vi "SetClassInstance.vi"(11 "OsciloscopioName":string) -> (3 "specific class reference":refnum<class "Osciloscope.lvclass">)   [LabVIEW 2020]
uses:
  Classes/Implementations/Osciloscope/Osciloscope.lvclass
  Classes/Implementations/TektronicsTDS/TektroniksTDS.lvclass
  C:/Users/HP/Documents/7mo/Instrumentacion/Parcial2/Osciloscope/Osciloscopio_DuranMu-oz/OsciloscopioProject/Classes/Implementations/Osciloscope/Osciloscope.lvclass
  Classes/Implementations/Keysight/Keysight.lvclass
panel:
  out "OsciloscopeName":refnum<class "Osciloscope.lvclass">
  in  "TypeOsciloscope":string
  out "Classes":string[](array[string])
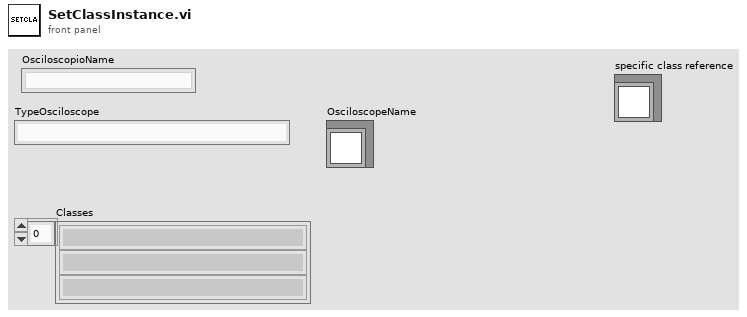
[diagram p1: front panel]
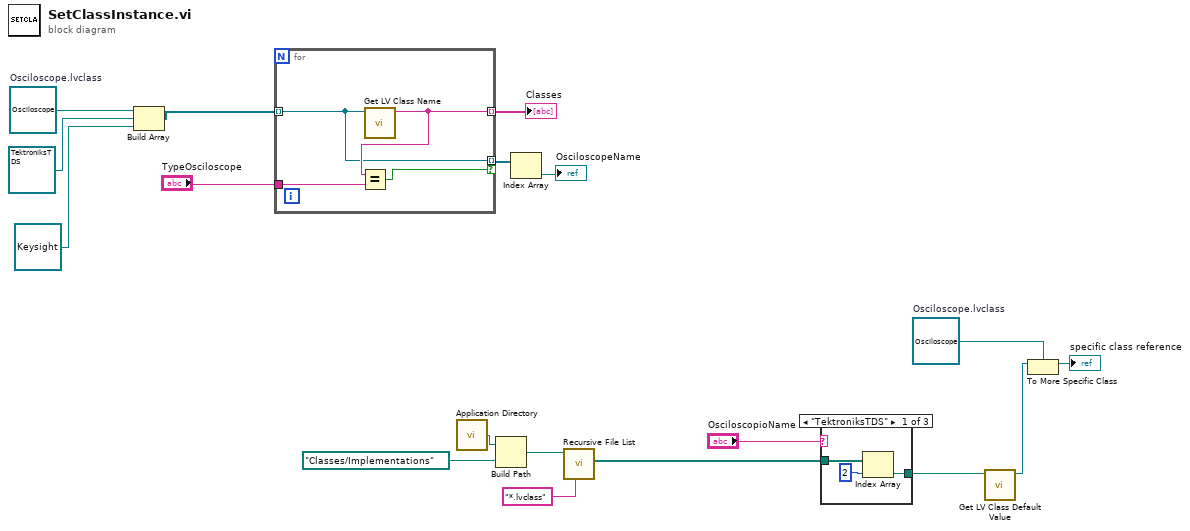
[diagram p0: block diagram]
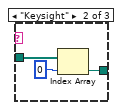
[diagram p2: hidden frame]
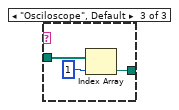
[diagram p3: hidden frame]
diagram:
  w3 = refnum<class "Osciloscope.lvclass"> refnum  # Osciloscope.lvclass
  w14 = refnum<class "Osciloscope.lvclass"> refnum  # Osciloscope.lvclass
  n1 = Build Array(w14, refnum<class "TektroniksTDS.lvclass"> refnum ("TektroniksTDS.lvclass"), refnum<class "Keysight.lvclass"> refnum ("Keysight.lvclass")) -> (w15:refnum<class "Osciloscope.lvclass">[])
  n2 = for {
    tunnel: w15 -> [w20] mode=indexing
    tunnel: [w21] -> w18 mode=indexing
    tunnel: "TypeOsciloscope" -> [w22]
    tunnel: [w20] -> w16 mode=indexing if=w19
    n3 = call <vilib>:"Get LV Class Name.vi"("object"=w20) -> ("class name"=w21:string)  [unwired: 9 in, 1 out]
    n4 = Equal?(x=w21, y=w22) -> (x = y?=w19:bool)
  }
  "Classes" <- w18
  n5 = call <vilib>:"Application Directory.vi"() -> ("Application Directory"=w9:path)
  n6 = Build Path(base path=w9, name or relative path=path "Classes/Implementations") -> (appended path=w7:path)
  n7 = Index Array(array=w16) -> (element=→"OsciloscopeName":refnum<class "Osciloscope.lvclass">)  [unwired: 1 in]
  n8 = call <vilib>:"Recursive File List.vi"("pattern"="*.lvclass", "Folder Path"=w7) -> ("All Files in Dir"=w10:path[])  [unwired: 5 in, 4 out]
  n9 = case shown="\"TektroniksTDS\"" "OsciloscopioName" {
    tunnel: w10 -> [w25 w28 w31]
    tunnel: [w23 w26 w30] -> w5
    frame "TektroniksTDS" {
      n10 = Index Array(array=w25, index=2) -> (element=w23:path)
    }
    frame "Keysight" {
      n11 = Index Array(array=w28, index=0) -> (element=w26:path)
    }
    frame "Osciloscope", Default {
      n12 = Index Array(array=w31, index=1) -> (element=w30:path)
    }
  }
  n13 = call <vilib>:"Get LV Class Default Value.vi"("class path"=w5) -> ("object"=w4:refnum<class>)  [unwired: 9 in, 1 out]
  n14 = To More Specific Class(target class=w3, reference=w4) -> (specific class reference=→"specific class reference":refnum<class "Osciloscope.lvclass">)  [unwired: 1 in, 1 out]
